vi "Refresh Auth.vi"(8 "error in (no error)":errorcluster, 9 "Timeout S (60)":dbl=60.0, 10 "Authorization in":refnum<class "Authorization.lvclass">, 11 "OAuth2 in":refnum<class "OAuth2.lvclass">) -> (0 "error out":errorcluster, 1 "Async Authentication":refnum<class "Async Authorization.lvclass">, 3 "OAuth2 out":refnum<class "OAuth2.lvclass">)   [LabVIEW 2020, in "OAuth2.lvlib" / "OAuth2.lvclass"]
uses:
  OAuth2.lvclass
  OAuth2.lvclass/OAuth2.ctl
  Authorization/Authorization.lvclass
  Async Authorization/Async Authorization.lvclass
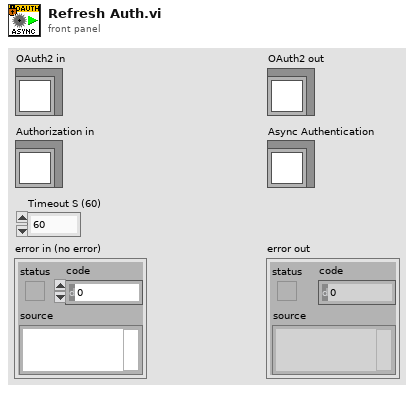
[diagram p1: front panel]
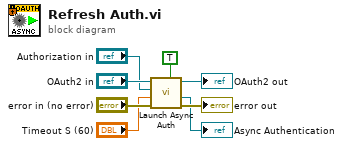
[diagram p0: block diagram]
diagram:
  n1 = call "Launch Async Auth.vi"("Refresh Only?"=TRUE, "error in (no error)"="error in (no error)", "Timeout S (60)"="Timeout S (60)", "Authorization in"="Authorization in", "OAuth2 in"="OAuth2 in") -> ("error out"=→"error out":errorcluster, "Async Authentication"=→"Async Authentication":refnum<class "Async Authorization.lvclass">, "OAuth2 out"=→"OAuth2 out":refnum<class "OAuth2.lvclass">)  [unwired: 4 in]
